vi "bboxsubvi.vi"(0 "Image":T1, 1 "size":dbl, 2 "def num":i32, 3 "array":dbl[][](array[numeric]), 4 "Drawing Mode (Frame)":u32(ring)=1 items=["Frame", "Fill"], 5 "error in":errorcluster) -> (14 "Image Out":T1, 19 "error out":errorcluster)   [LabVIEW 2019]
uses:
  <vilib>/vision/Image Controls.llb/IMAQ Image.ctl
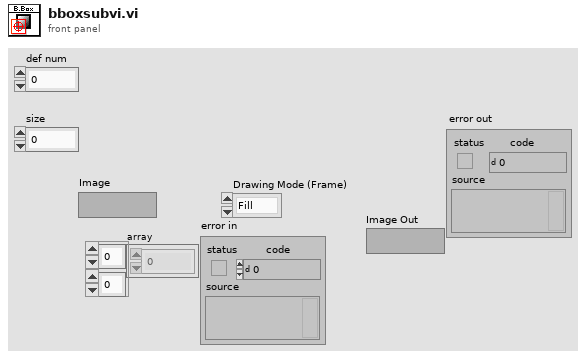
[diagram p1: front panel]
types:
  T1 = typedef "IMAQ Image.ctl" = refnum<image>
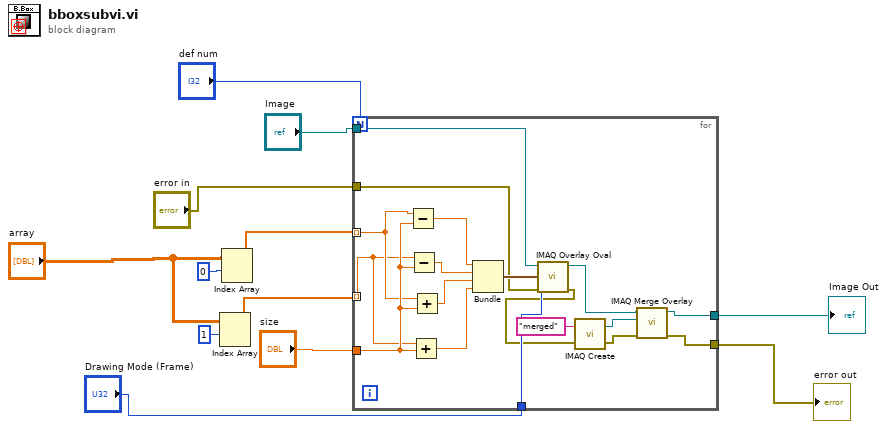
[diagram p0: block diagram]
diagram:
  n1 = Index Array(array="array", index (row)=1) -> (element=w9:dbl[])  [unwired: 1 in]
  n2 = Index Array(array="array", index (row)=0) -> (element=w10:dbl[])  [unwired: 1 in]
  n3 = for {
    N: "def num" -> [_]
    tunnel: "size" -> [w30]
    tunnel: w10 -> [w26] mode=indexing
    tunnel: w9 -> [w25] mode=indexing
    tunnel: "Image" -> [w22]
    tunnel: "Drawing Mode (Frame)" -> [w21]
    tunnel: [w15] -> w5
    tunnel: [w14] -> w4
    tunnel: "error in" -> [w13]
    n4 = Subtract(x=w26, y=w30) -> (x-y=w29:dbl)
    n5 = Subtract(x=w25, y=w30) -> (x-y=w27:dbl)
    n6 = Add(x=w25, y=w30) -> (x+y=w23:dbl)
    n7 = Add(x=w26, y=w30) -> (x+y=w24:dbl)
    n8 = Bundle(w29, w27, w24, w23) -> (w28:cluster{dbl, dbl, dbl, dbl})  [unwired: 1 in]
    n9 = call "IMAQ Overlay Oval"("error in (no error)"=w13, "Drawing Mode (Frame)"=w21, "Bounding Rectangle"=w28, "Image"=w22) -> ("error out"=w19:errorcluster, "Image Out"=w18:T1)  [unwired: 6 in]
    n10 = call "IMAQ Create"("Image Name"="merged", "error in (no error)"=w19) -> ("New Image"=w17:T1, "error out"=w16:errorcluster)  [unwired: 3 in]
    n11 = call "IMAQ Merge Overlay"("error in (no error)"=w16, "Image Dst"=w17, "Image Src"=w18) -> ("error out"=w15:errorcluster, "Image Dst Out"=w14:T1)  [unwired: 7 in]
  }
  "Image Out" <- w4
  "error out" <- w5
